vi "Labview's 8-bit color.vi"() -> ()   [LabVIEW 2009]
uses:
  <vilib>/picture/picture.llb/Draw 8-Bit Pixmap.vi
panel:
  in  "stop":bool
  out "Boolean array":bool[](array[boolean])
  out "Picture":picture
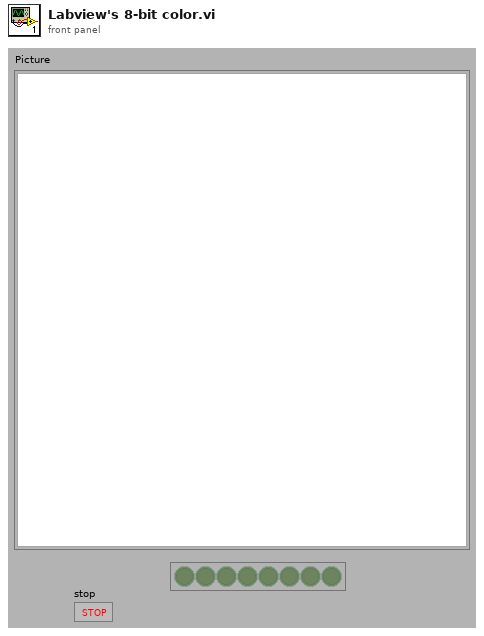
[diagram p1: front panel]
types:
  T1 = typedef "LVMouseTypeDef.ctl" = cluster{"Mouse Position":cluster{"X":i32, "Y":i32}, "Mouse Modifiers":cluster{"Button Down":bool, "Shift Mod":bool, "Menu Mod":bool, "Option Mod":bool}}
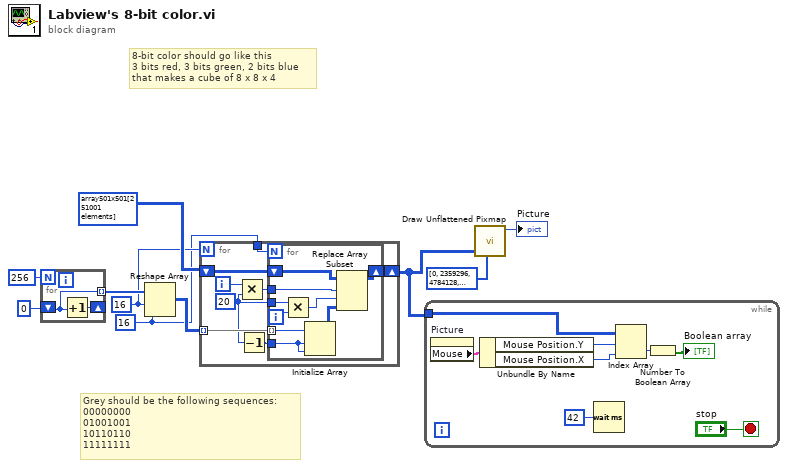
[diagram p0: block diagram]
diagram:
  w2 = 16 ("dimension size")
  w6 = 16 ("dimension size")
  # "Grey should be the following sequences:\n00000000\n01001001\n10110110\n11111111"
  # "8-bit color should go like this\n3 bits red, 3 bits green, 2 bits blue\nthat makes a cube of 8 x 8 x 4"
  n1 = for {
    N: 256 -> [_]
    shift-right: [w12] -> _
    shift-left: u8 0 ("Numeric") -> [w11]
    tunnel: [w11] -> w9 mode=indexing
    n2 = Increment(x=w11) -> (x+1=w12:u8)
  }
  n3 = Reshape Array(w9, w6, w2) -> (w7:u8[][])
  n4 = for {
    N: w6 -> [_]
    tunnel: w7 -> [w18] mode=indexing
    shift-right: [w19] -> w4
    shift-left: u8[][] array501x501[251001 elements] ("array") -> [w20]
    tunnel: w2 -> [w14]
    i -> [w17]
    w15 = 20 ("y")
    n5 = Multiply(x=w17, y=w15) -> (x*y=w16:i32)
    n6 = Decrement(x=w15) -> (x-1=w13:i32)
    n7 = for {
      N: w14 -> [_]
      tunnel: w18 -> [w24] mode=indexing
      tunnel: w16 -> [w27]
      tunnel: w15 -> [w25]
      tunnel: w13 -> [w23]
      shift-right: [w28] -> w19
      shift-left: w20 -> [w29]
      i -> [w26]
      n8 = Multiply(x=w25, y=w26) -> (x*y=w22:i32)
      n9 = Initialize Array(w24, w23, w23) -> (w21:u8[][])
      n10 = Replace Array Subset(array=w29, new element=w21, index (row)=w27, index (col)=w22) -> (w28:u8[][])
    }
  }
  n11 = while {
    tunnel: w4 -> [w36]
    stop <- "stop" stop-if-true
    n12 = property on="Picture" class="Pict"() -> ("Mouse"=w37:T1)  [unwired: 2 in, 2 out]
    n13 = Unbundle By Name(w37) -> ("Mouse Position.Y"=w35:i32, "Mouse Position.X"=w34:i32)
    n14 = Wait (ms)(milliseconds to wait=u32 42) -> ()  [unwired: 1 out]
    n15 = Index Array(array=w36, index (row)=w35, index (col)=w34) -> (element=w33:u8)
    n16 = Number To Boolean Array(number=w33) -> (Boolean array=→"Boolean array":bool[])
  }
  n17 = call-poly <vilib>:"Draw Unflattened Pixmap.vi"("data"=w4, "color table"=u32[] [0, 2359296, 4784128, 7143424, 9568256, 11927552, 14352384, 16711680, 9216, 2368512, 4793344, 7152640, 9577472, 11936768, 14361600, 16720896, 18688, 2377984, 4802816, 7162112, 9586944, 11946240, 14371072, 16730368, 27904, 2387200, 4812032, 7171328, 9596160, 11955456, 14380288, 16739584, 37376, 2396672, 4821504, 7180800, 9605632, 11964928, 14389760, 16749056, 46592, 2405888, 4830720, 7190016, 9614848, 11974144, 14398976, 16758272, 56064, 2415360, 4840192, 7199488, 9624320, 11983616, 14408448, 16767744, 65280, 2424576, 4849408, 7208704, 9633536, 11992832, 14417664, 16776960, 85, 2359381, 4784213, 7143509, 9568341, 11927637, 14352469, 16711765, 9301, 2368597, 4793429, 7152725, 9577557, 11936853, 14361685, 16720981, 18773, 2378069, 4802901, 7162197, 9587029, 11946325, 14371157, 16730453, 27989, 2387285, 4812117, 7171413, 9596245, 11955541, 14380373, 16739669, 37461, 2396757, 4821589, 7180885, 9605717, 11965013, 14389845, 16749141, 46677, 2405973, 4830805, 7190101, 9614933, 11974229, 14399061, 16758357, 56149, 2415445, 4840277, 7199573, 9624405, 11983701, 14408533, 16767829, 65365, 2424661, 4849493, 7208789, 9633621, 11992917, 14417749, 16777045, 170, 2359466, 4784298, 7143594, 9568426, 11927722, 14352554, 16711850, 9386, 2368682, 4793514, 7152810, 9577642, 11936938, 14361770, 16721066, 18858, 2378154, 4802986, 7162282, 9587114, 11946410, 14371242, 16730538, 28074, 2387370, 4812202, 7171498, 9596330, 11955626, 14380458, 16739754, 37546, 2396842, 4821674, 7180970, 9605802, 11965098, 14389930, 16749226, 46762, 2406058, 4830890, 7190186, 9615018, 11974314, 14399146, 16758442, 56234, 2415530, 4840362, 7199658, 9624490, 11983786, 14408618, 16767914, 65450, 2424746, 4849578, 7208874, 9633706, 11993002, 14417834, 16777130, 255, 2359551, 4784383, 7143679, 9568511, 11927807, 14352639, 16711935, 9471, 2368767, 4793599, 7152895, 9577727, 11937023, 14361855, 16721151, 18943, 2378239, 4803071, 7162367, 9587199, 11946495, 14371327, 16730623, 28159, 2387455, 4812287, 7171583, 9596415, 11955711, 14380543, 16739839, 37631, 2396927, 4821759, 7181055, 9605887, 11965183, 14390015, 16749311, 46847, 2406143, 4830975, 7190271, 9615103, 11974399, 14399231, 16758527, 56319, 2415615, 4840447, 7199743, 9624575, 11983871, 14408703, 16767999, 65535, 2424831, 4849663, 7208959, 9633791, 11993087, 14417919, 16777215] ("output array 2")) -> ("new picture"=→"Picture":picture)  [unwired: 7 in]
